vi "Create ODE.vi"(8 "error in (no error)":errorcluster, 9 "Body In":refnum<k20>, 10 "SimulatorEngine in":refnum<class "ODESimulator_Engine.lvclass">, 11 "Base in":refnum<class "ODESimulator_LinearConveyor.lvclass">) -> (0 "error out":errorcluster, 1 "Geom Out":refnum<k20>, 2 "SimulatorEngine out":refnum<class "ODESimulator_Engine.lvclass">, 3 "Base out":refnum<class "ODESimulator_LinearConveyor.lvclass">)   [LabVIEW 2017, in "NI_Robotics_Simulator.lvlib" / "ODESimulator_LinearConveyor.lvclass"]
uses:
  <vilib>/robotics/Simulator/Robot Factory/Conveyor/Linear/ODESimulator_LinearConveyor.lvclass
  <vilib>/robotics/Simulator/Engine/ODESimulator_Engine.lvclass
  <vilib>/robotics/Simulator/Robot Factory/Conveyor/Linear/ODESimulator_LinearConveyor.lvclass/ODESimulator_LinearConveyor.ctl
  <vilib>/robotics/Simulator/LVODE/Open Reference (Linear Conveyor).vi
  <vilib>/robotics/Simulator/LVODE/Open Reference (Box).vi
  <vilib>/robotics/Simulator/Robot Factory/Conveyor/Base/ODESimulator_Base_Conveyor.lvclass
  <resource>/objmgr/LVODE.rc
  <vilib>/robotics/Simulator/NI_Robotics_Simulator.lvlib
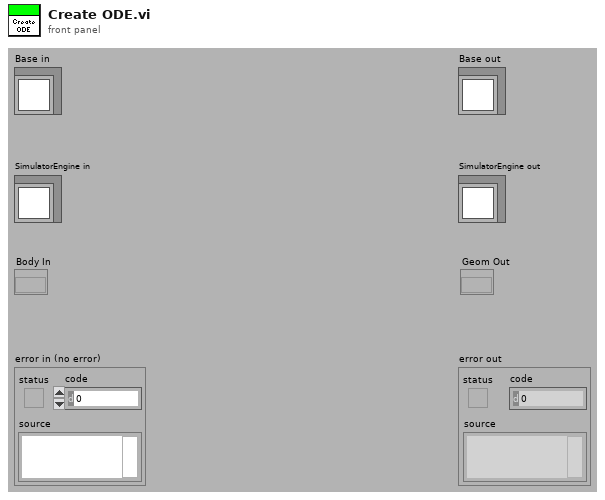
[diagram p1: front panel]
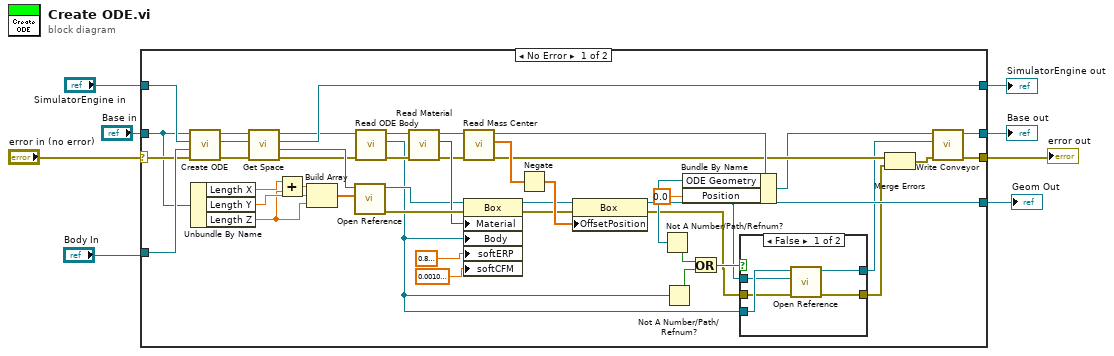
[diagram p0: block diagram]
diagram:
  n1 = case shown="No Error" "error in (no error)" {
    selector: "error in (no error)" -> [w37 w59]
    tunnel: [w17 w59] -> w1
    tunnel: [w16 w60] -> w4
    tunnel: "Base in" -> [w36 w60]
    tunnel: "SimulatorEngine in" -> [w49 w61]
    tunnel: [w48 w61] -> w3
    tunnel: [w20 _] -> w2
    tunnel: "Body In" -> [w47 _]
    frame No Error {
      n2 = call-parent "Create ODE.vi"("error in (no error)"=w37, "Body In"=w47, "SimulatorEngine in"=w49, "Base in"=w36) -> ("error out"=w52:errorcluster, "SimulatorEngine out"=w50:refnum<class "ODESimulator_Engine.lvclass">, "Base out"=w51:refnum<class "ODESimulator_LinearConveyor.lvclass">)  [unwired: 4 in, 1 out]
      n3 = Unbundle By Name(w36) -> ("Length X"=w11:sgl, "Length Y"=w44:sgl, "Length Z"=w10:sgl)
      n4 = call-dynamic "Get Space.vi"("error in (no error)"=w52, "SimulatorEngine in"=w50, "3D_Physics_Base in"=w51) -> ("error out"=w35:errorcluster, "Space"=w38:refnum<k20>, "SimulatorEngine out"=w48:refnum<class "ODESimulator_Engine.lvclass">, "3D_Physics_Base out"=w34:refnum<class "ODESimulator_LinearConveyor.lvclass">)  [unwired: 5 in]
      n5 = Add(x=w11, y=w10) -> (x+y=w9:sgl)
      n6 = Build Array(w9, w44, w10) -> (w45:sgl[])
      n7 = call-poly <vilib>:"Open Reference.vi"("Length"=w45, "Space In"=w38) -> ("error out"=w46:errorcluster, "Box Out"=w33:refnum<k20>)  [unwired: 8 in]
      n8 = call-dynamic "Read ODE Body.vi"("error in (no error)"=w35, "Base in"=w34) -> ("error out"=w39:errorcluster, "ODE Body"=w21:refnum<k20>, "Base out"=w40:refnum<class "ODESimulator_LinearConveyor.lvclass">)  [unwired: 7 in]
      n9 = call-dynamic "Read Material.vi"("error in (no error)"=w39, "Base in"=w40) -> ("error out"=w30:errorcluster, "Material"=w41:u16, "Base out"=w29:refnum<class "ODESimulator_LinearConveyor.lvclass">)  [unwired: 7 in]
      n10 = call-dynamic "Read Mass Center.vi"("error in (no error)"=w30, "3D_Physics_Base in"=w29) -> ("error out"=w25:errorcluster, "Mass Center"=w32:sgl[], "3D_Physics_Base out"=w26:refnum<class "ODESimulator_LinearConveyor.lvclass">)  [unwired: 7 in]
      n11 = property class="Box"(reference=w33, error in=w46, "Material"=w41, "Body"=w21, "softERP"=sgl 0.8 ("surface:soft ERP"), "softCFM"=sgl 0.001 ("surface:soft CFM")) -> (reference out=w28:refnum<k20>, error out=w27:errorcluster)
      n12 = Negate(x=w32) -> (-x=w31:sgl[])
      n13 = property class="Box"(reference=w28, error in=w27, "OffsetPosition"=w31) -> (reference out=w20:refnum<k20>, error out=w19:errorcluster)
      n14 = Not A Number/Path/Refnum?(number/path/refnum=w20) -> (NaN/Path/Refnum?=w24:bool)
      n15 = Not A Number/Path/Refnum?(number/path/refnum=w21) -> (NaN/Path/Refnum?=w23:bool)
      n16 = Bundle By Name(cluster=w26, "ODE Geometry"=w20, "Position"=0.0) -> (w18:refnum<class "ODESimulator_LinearConveyor.lvclass">)
      n17 = Or(x=w24, y=w23) -> (x .or. y?=w22:bool)
      n18 = case shown="False" w22 {
        tunnel: w21 -> [w57 _]
        tunnel: w20 -> [w56 _]
        tunnel: w19 -> [w55 w58]
        tunnel: [w54 _] -> w14
        tunnel: [w53 w58] -> w13
        frame False {
          n19 = call-poly <vilib>:"Open Reference.vi"("error in (no error)"=w55, "Geom"=w56, "Body"=w57) -> ("error out"=w53:errorcluster, "Conveyor"=w54:refnum<k20>)  [unwired: 7 in]
        }
        frame True {
        }
      }
      n20 = Merge Errors(w25, w13) -> (w15:errorcluster)
      n21 = call-dynamic "Write Conveyor.vi"("error in (no error)"=w15, "Conveyor"=w14, "ODESimulator_Base_Conveyor in"=w18) -> ("error out"=w17:errorcluster, "ODESimulator_Base_Conveyor out"=w16:refnum<class "ODESimulator_LinearConveyor.lvclass">)  [unwired: 7 in]
    }
    frame Error {
    }
  }
  "error out" <- w1
  "Base out" <- w4
  "SimulatorEngine out" <- w3
  "Geom Out" <- w2
